vi "PASV.vi"(8 "error in (no error)":errorcluster, 11 "FTP in":refnum<class "FTP.lvclass">) -> (0 "error out":errorcluster, 3 "FTP out":refnum<class "FTP.lvclass">)   [LabVIEW 2017, in "FTP_UpgradeCSMF.lvlib" / "FTP.lvclass"]
uses:
  FTP.lvclass
  FTP.lvclass/FTP.ctl
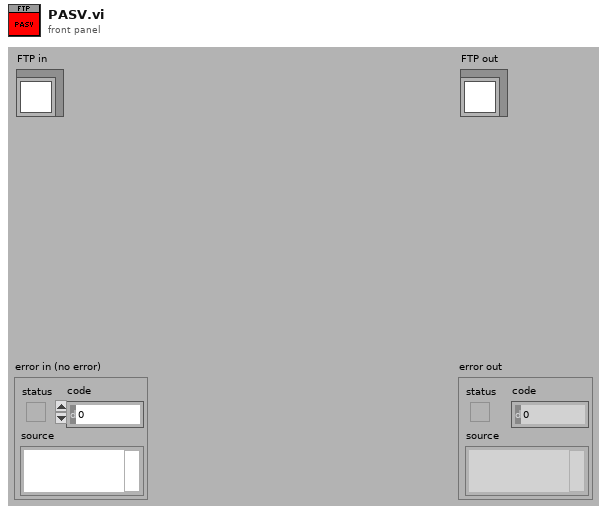
[diagram p1: front panel]
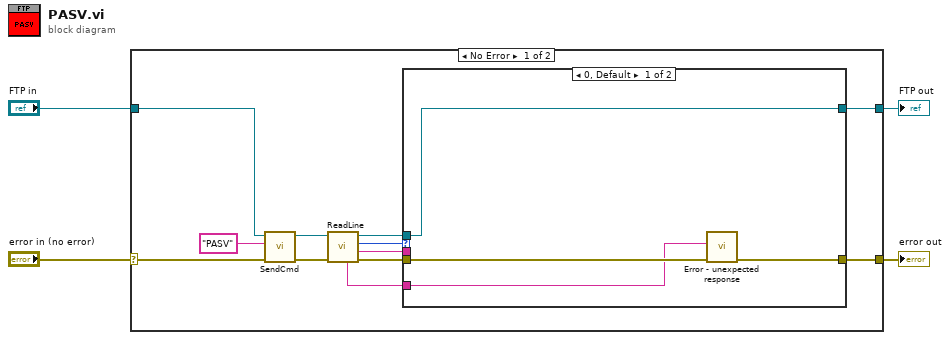
[diagram p0: block diagram]
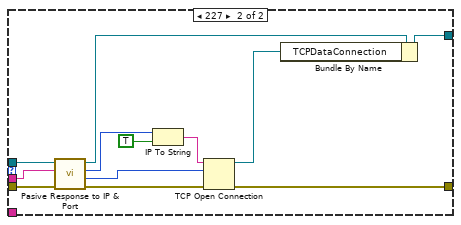
[diagram p2: hidden frame]
diagram:
  n1 = case shown="No Error" "error in (no error)" {
    selector: "error in (no error)" -> [w15 w34]
    tunnel: [w9 w34] -> w3
    tunnel: [w10 w33] -> w1
    tunnel: "FTP in" -> [w16 w33]
    frame No Error {
      n2 = call "SendCmd.vi"("error in (no error)"=w15, "cmd"="PASV", "FTP in"=w16) -> ("error out"=w13:errorcluster, "FTP out"=w14:refnum<class "FTP.lvclass">)  [unwired: 7 in]
      n3 = call "ReadLine.vi"("error in (no error)"=w13, "FTP in"=w14) -> ("error out"=w12:errorcluster, "Line"=w7:string, "code"=w8:i32, "FTP out"=w11:refnum<class "FTP.lvclass">, "Full Line"=w5:string)  [unwired: 5 in]
      n4 = case shown="0, Default" w8 {
        tunnel: w12 -> [w19 w32]
        tunnel: w11 -> [w20 w31]
        tunnel: [w20 w23] -> w10
        tunnel: [w17 w24] -> w9
        tunnel: w7 -> [_ w30]
        tunnel: w5 -> [w18 _]
        frame 0, Default {
          n5 = call "Error - unexpected response.vi"("error in (no error)"=w19, "Full Response"=w18) -> ("error out"=w17:errorcluster)  [unwired: 9 in]
        }
        frame 227 {
          n6 = call "Pasive Response to IP & Port.vi"("error in (no error)"=w32, "Response"=w30, "FTP in"=w31) -> ("error out"=w28:errorcluster, "Port"=w21:u16, "IP"=w26:u32, "FTP out"=w29:refnum<class "FTP.lvclass">)  [unwired: 5 in]
          n7 = IP To String(1:TRUE ("dot notation? (F)"), 2:w26) -> (0:w27:string)
          n8 = TCP Open Connection(address=w27, remote port or service name=w21, error in (no error)=w28) -> (connection ID=w22:refnum<k5>, error out=w24:errorcluster)  [unwired: 2 in]
          n9 = Bundle By Name(cluster=w29, "TCPDataConnection"=w22) -> (w23:refnum<class "FTP.lvclass">)
        }
      }
    }
    frame Error {
    }
  }
  "error out" <- w3
  "FTP out" <- w1
